vi "#8.vi"(0 "System no.":i32=1 min=1 max=4 step=1, 5 "error in":errorcluster) -> (14 "Macro running?":bool, 15 "String read":string, 19 "error out":errorcluster)   [LabVIEW 2020]
doc: "Sends ASCII #8 without Linefeed and returns Macro running? indicating whether a macro is running or not.\n\nE-816: This command cannot be issued to a slave. Check controller manual to find out if #8 is supported.\n\nC-887, F-206, M-8X0: Only for GCS syntax version = GCS 2.0 or higher (check with CSV?.vi. If CSV?.vi is not supported, syntax version is GCS 1.0)."
panel:
  # "Sends ASCII #8 without LineFeed and returns \"Macro running?\" indicating \nwhether a macro is running or not."
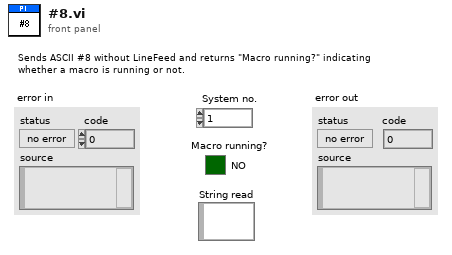
[diagram p1: front panel]
types:
  T1 = enum16{"Disable error check", "Force error check", "Use global settings"}
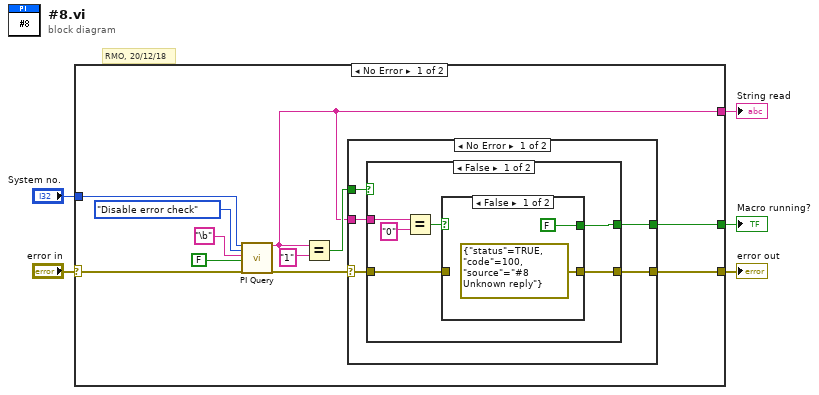
[diagram p0: block diagram]
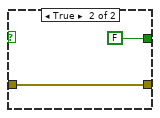
[diagram p2: hidden frame]
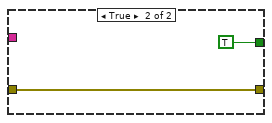
[diagram p3: hidden frame]
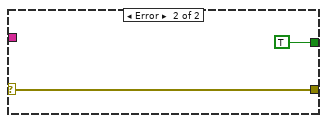
[diagram p4: hidden frame]
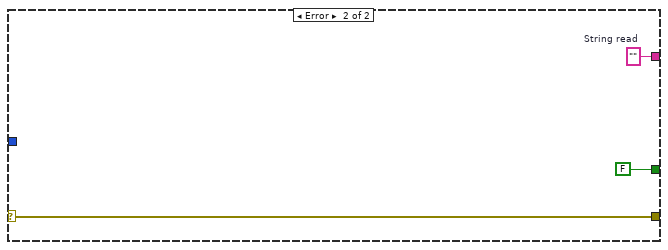
[diagram p5: hidden frame]
diagram:
  # "RMO, 20/12/18"
  n1 = case shown="No Error" "error in" {
    selector: "error in" -> [w9 w38]
    tunnel: "System no." -> [w15 _]
    tunnel: [w13 w38] -> w4
    tunnel: [w12 FALSE] -> w3
    tunnel: [w8 w36] -> w2
    frame No Error {
      n2 = call "PI Query.vi"("System no."=w15, "Error check settings"=T1."Disable error check", "String to send"="\b", "Attach termination char.?"=FALSE ("Attach Linefeed?"), "error in"=w9) -> ("String read"=w8:string, "error out"=w6:errorcluster)  [unwired: 2 in, 11 out]
      n3 = Equal?(x=w8, y="1" ("String read")) -> (x = y?=w14:bool)
      n4 = case shown="No Error" w6 {
        selector: w6 -> [w17 w34]
        tunnel: w14 -> [w21 _]
        tunnel: [w20 w34] -> w13
        tunnel: [w19 TRUE] -> w12
        tunnel: w8 -> [w18 _]
        frame No Error {
          n5 = case shown="False" w21 {
            tunnel: w17 -> [w24 w33]
            tunnel: [w23 w33] -> w20
            tunnel: [w25 TRUE] -> w19
            tunnel: w18 -> [w27 _]
            frame False {
              n6 = Equal?(x=w27, y="0" ("String read")) -> (x = y?=w26:bool)
              n7 = case shown="False" w26 {
                tunnel: [FALSE FALSE] -> w25
                tunnel: w24 -> [_ w30]
                tunnel: [errorcluster {"status"=TRUE, "code"=100, "source"="#8 Unknown reply"} ("error out") w30] -> w23
                frame False {
                }
                frame True {
                }
              }
            }
            frame True {
            }
          }
        }
        frame Error {
        }
      }
    }
    frame Error {
      w36 = ""  # String read
    }
  }
  "error out" <- w4
  "Macro running?" <- w3
  "String read" <- w2
